vi "Main v00a.vi"() -> ()   [LabVIEW 2017]
uses:
  Controles/Objetos.ctl
  <vilib>/addons/database/Connection.llb/Conn ObjectReference.ctl
  <vilib>/NI/AMC/Update Message Routing Info.vi
  <vilib>/NI/AMC/Create Multiple Messages.vi
  <vilib>/NI/AMC/Read Termination Message.vi
  <vilib>/NI/AMC/Create Single Message.vi
  <vilib>/NI/AMC/Send Message.vi
  <vilib>/NI/AMC/Globals.vi
  <vilib>/Utility/file.llb/Read Delimited Spreadsheet (string).vi
  Globals/Global.vi
  <vilib>/addons/database/Connection.llb/DB Tools Open Connec (Path).vi
  ALT irMonitor/Gobal/Global variables.vi
  <vilib>/addons/database/NI_Database_API.lvlib
  <vilib>/NI/AMC/AMC.lvlib
panel:
  out "BBDD":bool
  in  "Consulta":bool
  in  "Registrado":string
  in  "Cambiar de usuario":bool
  in  "Jiffy csv":path
  in  "Registrar":bool
  out "error out":errorcluster
  in  "Objetos":T1
  out "DataBase":bool
  # "Contabilizador"
  # "powered by"
  # "Contabilizador v00a"
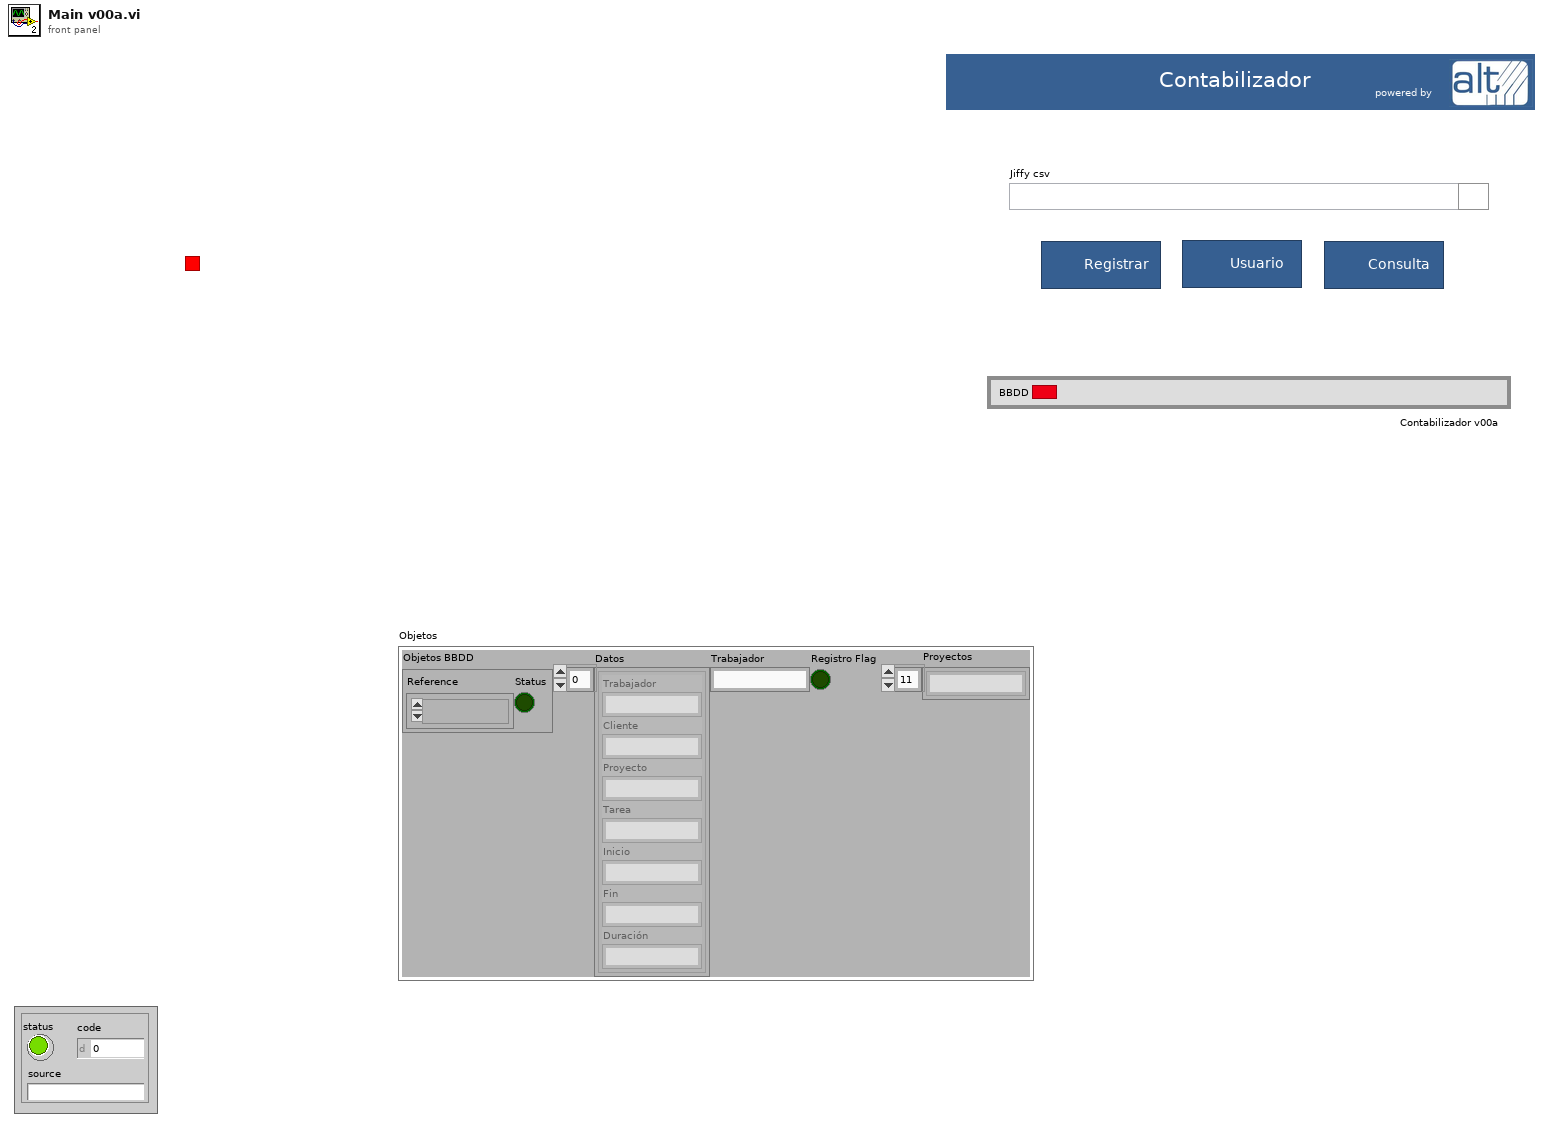
[diagram p1: front panel]
types:
  T1 = typedef "Objetos.ctl" = cluster{"Objetos BBDD":cluster{"Reference":T2, "Status":bool}, "Datos":cluster{"Trabajador":string, "Cliente":string, "Proyecto":string, "Tarea":string, "Inicio":string, "Fin":string, "Duración":string}[], "Trabajador":string, "Registro Flag":bool, "Proyectos":string[]}
  T2 = typedef "NI_Database_API.lvlib/Conn ObjectReference.ctl" = refnum<k1>
  T3 = typedef "AMC.lvlib/Message Queue.ctl" = refnum<queue>
  T4 = cluster{"Trabajador":string, "Cliente":string, "Proyecto":string, "Tarea":string, "Inicio":string, "Fin":string, "Duración":string}
  T5 = cluster{"Nombre de usuario":string, "Contraseña":string, "Trabajador":string}[]
  T6 = cluster{"Trabajador":string, "Cliente":string, "Proyecto":string, "Tarea":string, "Inicio":string, "Fin":string, "Duración":string}[]
  T7 = cluster{"Trabajador":string, "Cliente":string, "Proyecto":string, "Tarea":string, "Inicio":string, "Fin":string, i32}
  T8 = cluster{"Principal":string, "Base de datos":string, "Dialogs":string, "Log":string, "Cam 1":string, "Cam 2":string, "Cam 3":string, "Cam 4":string, "ioLogik":string}
  T9 = cluster{"Nombre":void, "Min":void, "Avg":void, "Max":void, "Condición":void, "Resultado":void, "date/time string":string}
  T10 = cluster{"Database UDL":path, "Settings":path, "Ports":path, "Log Events":path}
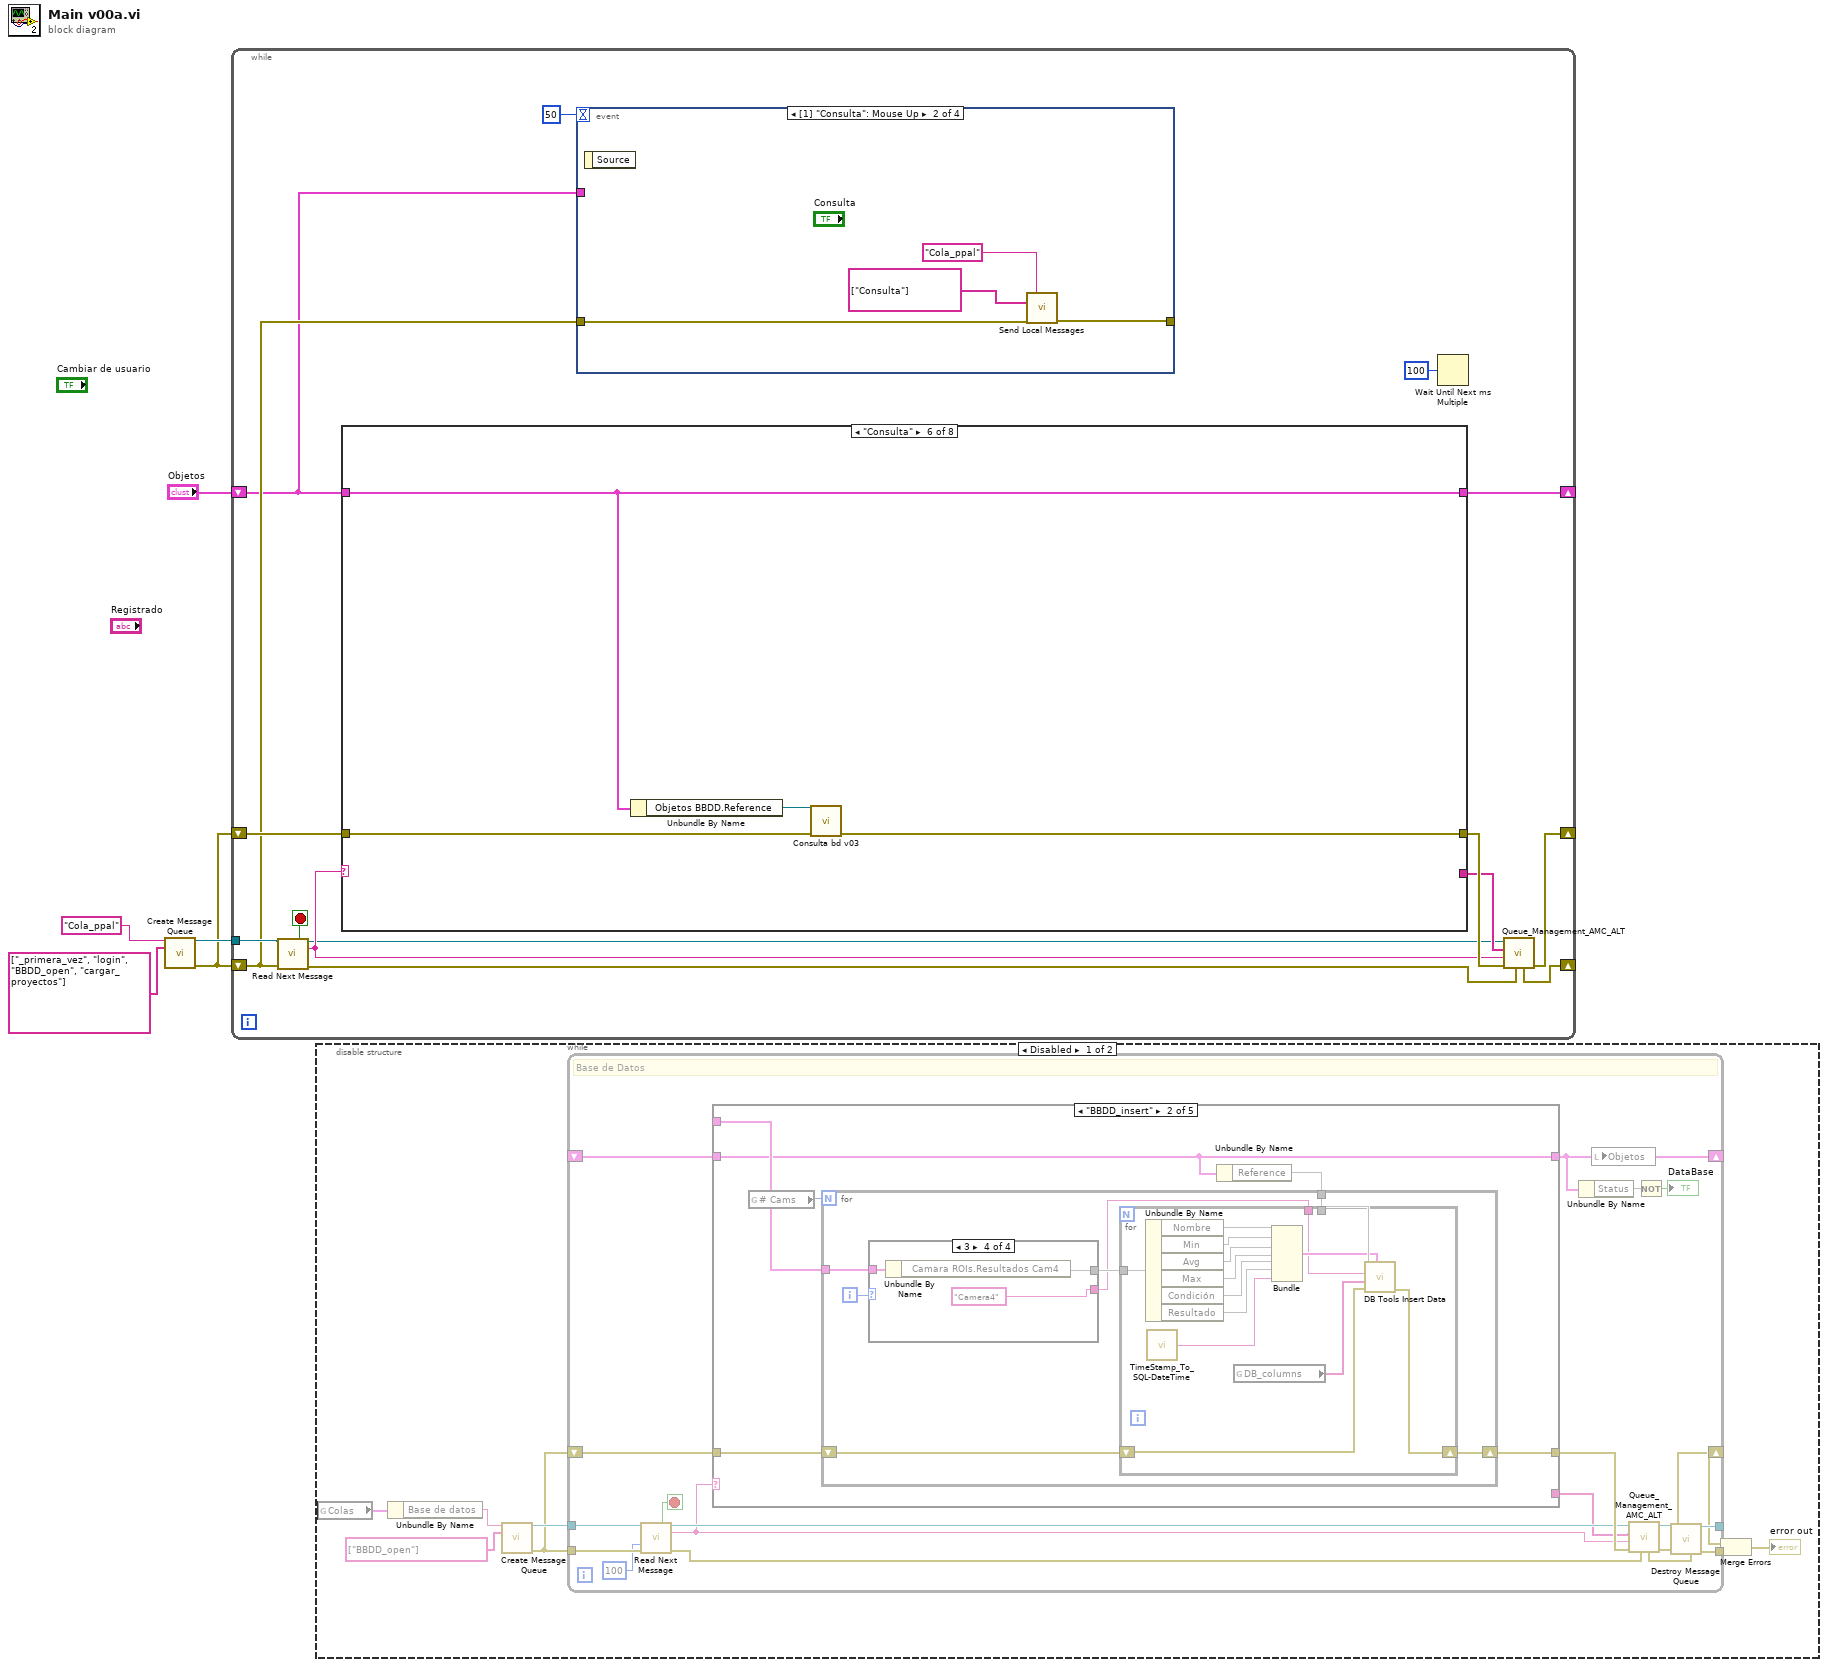
[diagram p0: block diagram]
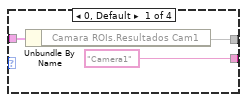
[diagram p3: hidden frame]
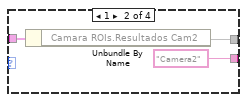
[diagram p4: hidden frame]
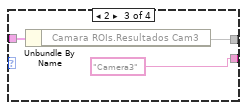
[diagram p5: hidden frame]
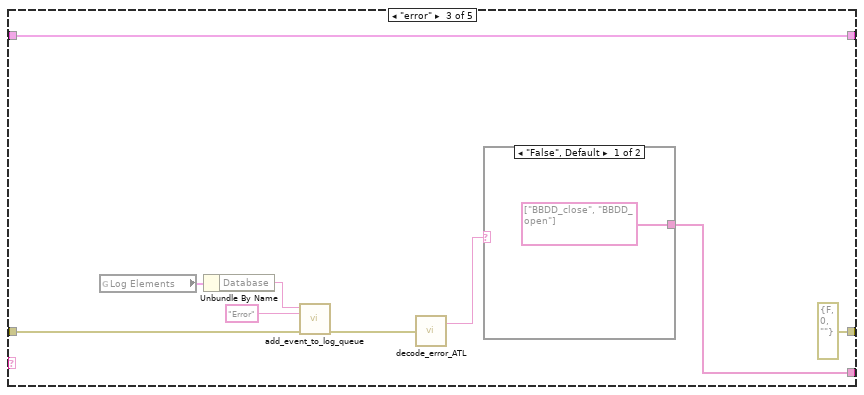
[diagram p6: hidden frame]
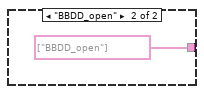
[diagram p7: hidden frame]
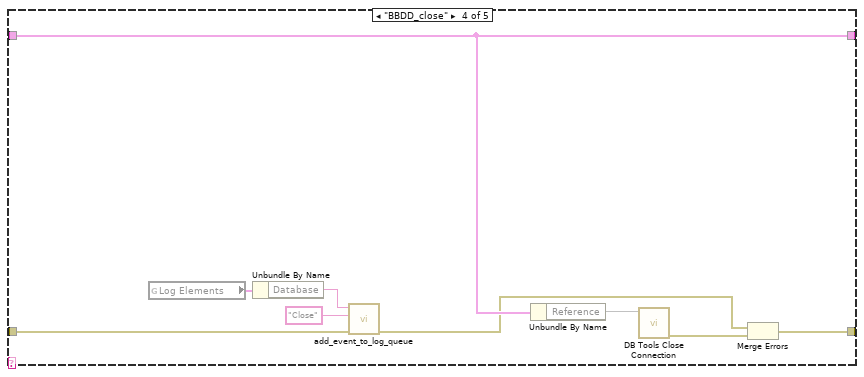
[diagram p8: hidden frame]
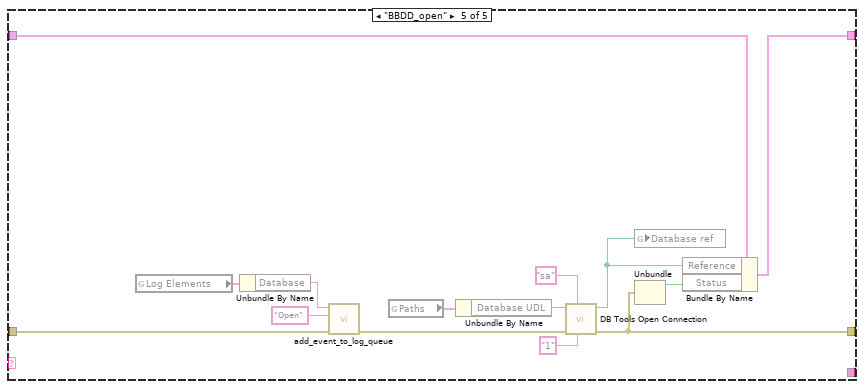
[diagram p9: hidden frame]
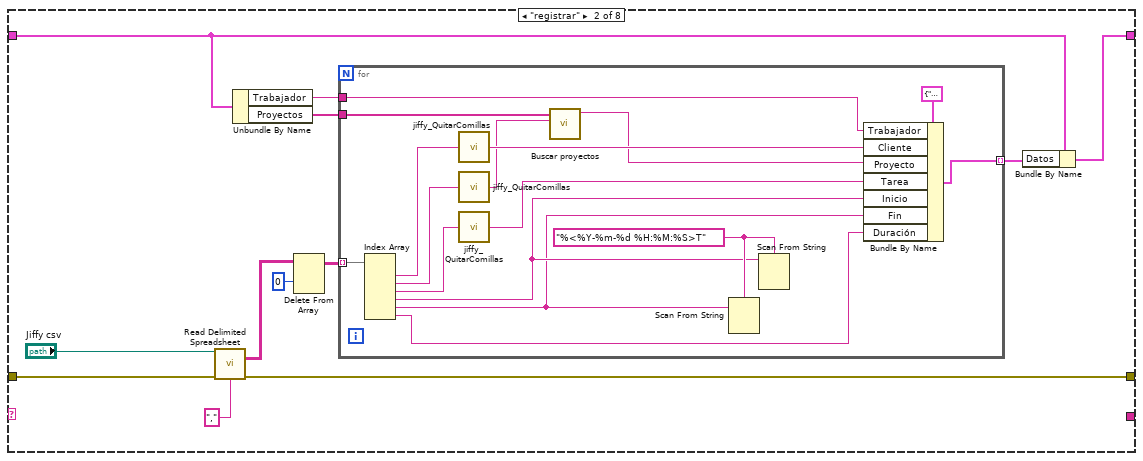
[diagram p12: hidden frame]
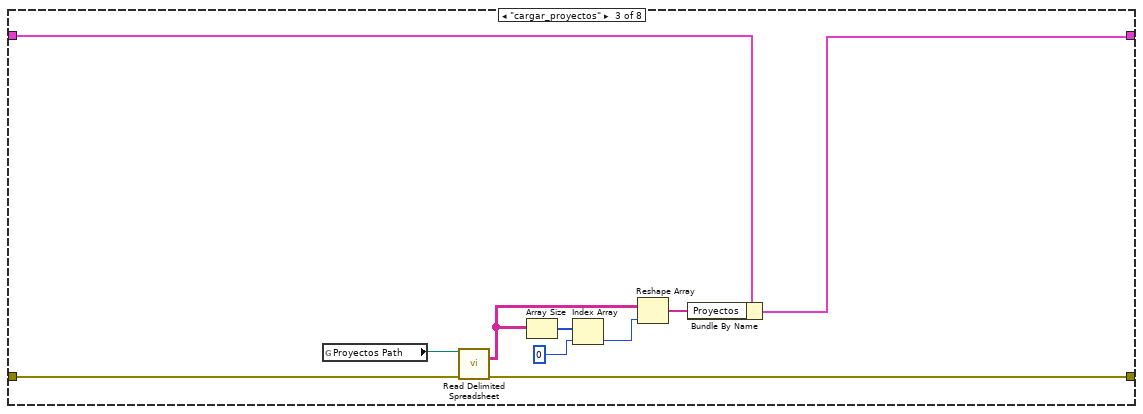
[diagram p13: hidden frame]
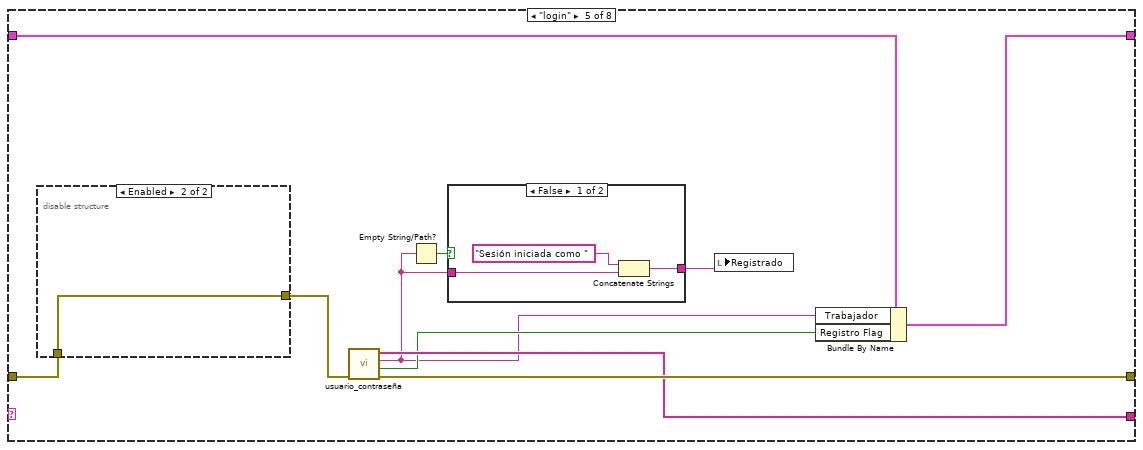
[diagram p15: hidden frame]
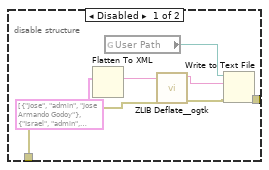
[diagram p16: hidden frame]
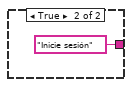
[diagram p17: hidden frame]
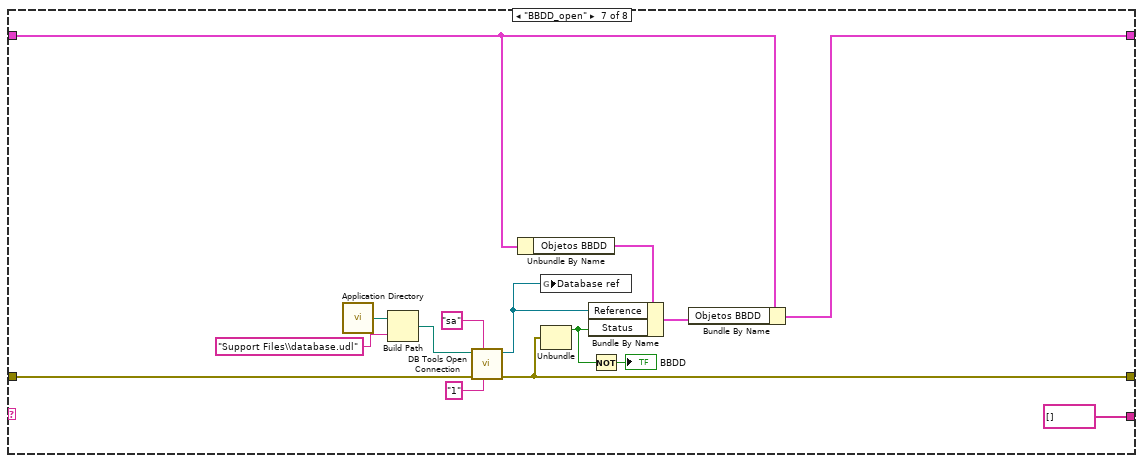
[diagram p18: hidden frame]
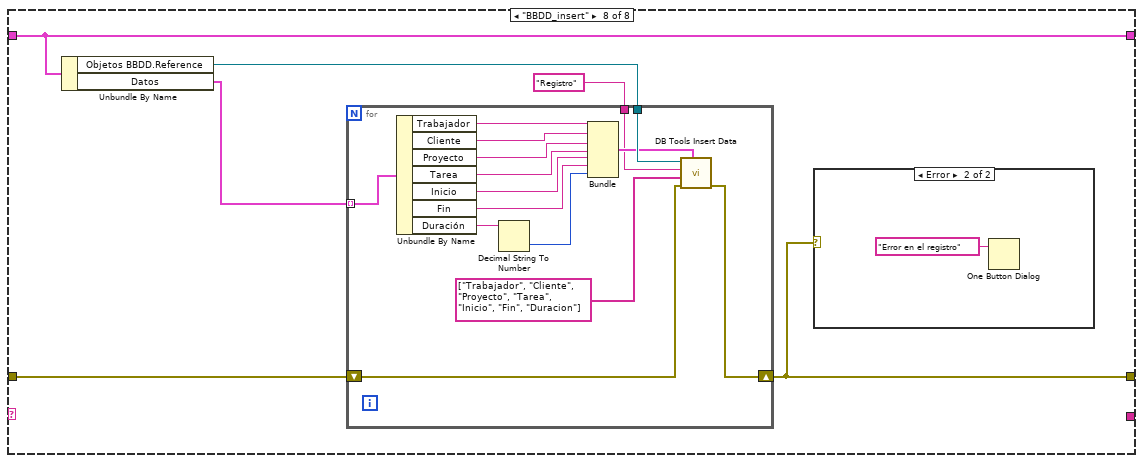
[diagram p19: hidden frame]
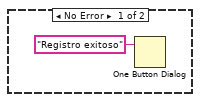
[diagram p20: hidden frame]
diagram:
  n1 = call <vilib>:"Create Message Queue.vi"("message queue name"="Cola_ppal", "initial message names"=string[] ["_primera_vez", "login", "BBDD_open", "cargar_proyectos"]) -> ("message queue out"=w4:T3, "error out"=w1:errorcluster)  [unwired: 12 in]
  n2 = while {
    shift-right: [w17] -> _
    shift-left: w1 -> [w9]
    tunnel: w4 -> [w19]
    shift-right: [w16] -> _
    shift-left: "Objetos" -> [w7]
    shift-right: [w13] -> _
    shift-left: w1 -> [w14]
    stop <- w20 stop-if-true
    n3 = call <vilib>:"Read Next Message.vi"("message queue in"=w19, "error in"=w9) -> ("exit process?"=w20:bool, "message queue out"=w10:T3, "message name"=w11:string, "error out"=w18:errorcluster)  [unwired: 6 in, 4 out]
    n4 = case shown="\"Consulta\"" w11 {
      tunnel: w7 -> [w21 w29 w56 w61 w68 w85 w96 w107]
      tunnel: [w21 w33 w55 w61 w67 w85 w95 w107] -> w16
      tunnel: w14 -> [_ w32 w59 w60 w71 w87 w94 w108]
      tunnel: [_ w31 w58 w60 w70 w86 w93 w103] -> w15
      tunnel: [_ _ _ _ w66 _ string[] [] ("Elementos a cola") _] -> w12
      frame "False", Default {
      }
      frame "registrar" {
        n5 = call-poly <vilib>:"Read Delimited Spreadsheet.vi"("file path (dialog if empty)"="Jiffy csv", "error in (no error)"=w32, "delimiter (\\t)"="," ("delimiter (\\t)")) -> ("all rows"=w27:string[][], "error out"=w31:errorcluster)  [unwired: 7 in, 4 out]
        n6 = Unbundle By Name(w29) -> ("Trabajador"=w23:string, "Proyectos"=w22:string[])
        n7 = Delete From Array(array=w27, index (row)=0) -> (array with subset deleted=w26:string[][])  [unwired: 2 in, 1 out]
        n8 = for {
          tunnel: w26 -> [w49] mode=indexing
          tunnel: [w39] -> w24 mode=indexing
          tunnel: w23 -> [w37]
          tunnel: w22 -> [w35]
          w46 = "%<%Y-%m-%d %H:%M:%S>T" ("format string")
          n9 = Index Array(array=w49) -> (element #1=w45:string, element #2=w48:string, element #3=w47:string, element #4=w41:string, element #5=w40:string, element #6=w38:string)  [unwired: 6 in]
          n10 = call "jiffy_QuitarComillas.vi"("String in"=w45) -> ("String out"=w43:string)
          n11 = call "jiffy_QuitarComillas.vi"("String in"=w48) -> ("String out"=w36:string)
          n12 = call "jiffy_QuitarComillas.vi"("String in"=w47) -> ("String out"=w42:string)
          n13 = call "Buscar proyectos.vi"("String out"=w36, "Proyectos"=w35) -> ("Proyecto"=w34:string)  [unwired: 9 in]
          n14 = Scan From String(format string=w46, input string=w40) -> ()  [unwired: 4 in, 3 out]
          n15 = Scan From String(format string=w46, input string=w41) -> ()  [unwired: 4 in, 3 out]
          n16 = Bundle By Name(cluster=T4 {"Trabajador"="", "Cliente"="", "Proyecto"="", "Tarea"="", "Inicio"="", "Fin"="", "Duración"=""} ("Cluster"), "Trabajador"=w37, "Cliente"=w43, "Proyecto"=w34, "Tarea"=w42, "Inicio"=w41, "Fin"=w40, "Duración"=w38) -> (w39:T4)
        }
        n17 = Bundle By Name(cluster=w29, "Datos"=w24) -> (w33:T1)
      }
      frame "cargar_proyectos" {
        n18 = global read "Global.vi" "Proyectos Path"() -> (w57:path)
        n19 = call-poly <vilib>:"Read Delimited Spreadsheet.vi"("file path (dialog if empty)"=w57, "error in (no error)"=w59) -> ("all rows"=w53:string[][], "error out"=w58:errorcluster)  [unwired: 8 in, 4 out]
        n20 = Array Size(array=w53) -> (size(s)=w52:i32[])
        n21 = Index Array(array=w52, index=0) -> (element=w50:i32)
        n22 = Reshape Array(w53, w50) -> (w54:string[])
        n23 = Bundle By Name(cluster=w56, "Proyectos"=w54) -> (w55:T1)
      }
      frame "_primera_vez" {
      }
      frame "login" {
        n24 = disable-structure shown="Enabled" {
          disable-tunnel: w71 -> [w78 w79]
          disable-tunnel: [w77 w79] -> w69
          frame Disabled {
            n25 = Flatten To XML(anything=T5 [{"Nombre de usuario"="Jose", "Contraseña"="admin", "Trabajador"="Jose Armando Godoy"}, {"Nombre de usuario"="Israel", "Contraseña"="admin", "Trabajador"="Israel Garcia"}, {"Nombre de usuario"="Alejandro", "Contraseña"="admin", "Trabajador"="Alejandro Ortiz"}, {"Nombre de usuario"="Jair", "Contraseña"="admin", "Trabajador"="Jair Paredes"}] ("Array")) -> (xml string=w73:string)
            n26 = global read "Global.vi" "User Path"() -> (w72:path)
            n27 = call <userlib>:"ZLIB Deflate__ogtk.vi"("error in (no error)"=w78, "input"=w73) -> ("error out"=w75:errorcluster, "deflated output"=w76:string)  [unwired: 3 in, 1 out]
            n28 = Write to Text File(file (use dialog)=w72, text=w76, error in=w75) -> (error out=w77:errorcluster)  [unwired: 1 in, 2 out]
          }
          frame Enabled {
          }
        }
        n29 = call "usuario_contraseña.vi"("error in"=w69) -> ("error out"=w70:errorcluster, "Registro Flag"=w65:bool, "Trabajador"=w62:string, "Elemento a cola"=w66:string[])  [unwired: 7 in]
        n30 = Empty String/Path?(string/path=w62) -> (empty?=w64:bool)
        n31 = case shown="False" w64 {
          tunnel: [w81 "Inicie sesión"] -> w63
          tunnel: w62 -> [w80 _]
          frame False {
            n32 = Concatenate Strings("Sesión iniciada como ", w80) -> (w81:string)
          }
          frame True {
          }
        }
        n33 = local write "Registrado"(w63) -> ()
        n34 = Bundle By Name(cluster=w68, "Trabajador"=w62, "Registro Flag"=w65) -> (w67:T1)
      }
      frame "Consulta" {
        n35 = Unbundle By Name(w85) -> ("Objetos BBDD.Reference"=w84:T2)
        n36 = call "Consulta bd v03.vi"("error in (no error)"=w87, "Database"=w84) -> ("error out"=w86:errorcluster)  [unwired: 9 in]
      }
      frame "BBDD_open" {
        n37 = call <vilib>:"Application Directory.vi"() -> ("Application Directory"=w92:path)
        n38 = Build Path(base path=w92, name or relative path="Support Files\\database.udl") -> (appended path=w90:path)
        n39 = call-poly <vilib>:"DB Tools Open Connection.vi"("password"="1", "userID"="sa", "error in (no error)"=w94, "connection information"=w90) -> ("error out"=w93:errorcluster, "connection reference"=w99:T2)  [unwired: 4 in]
        n40 = Unbundle By Name(w96) -> ("Objetos BBDD"=w98:cluster{"Reference":T2, "Status":bool})
        n41 = global write "Global variables.vi" "Database ref"(w99) -> ()
        n42 = Unbundle(w93) -> ("status"=w100:bool)  [unwired: 2 out]
        n43 = Bundle By Name(cluster=w98, "Reference"=w99, "Status"=w100) -> (w97:cluster{"Reference":T2, "Status":bool})
        n44 = Not(x=w100) -> (.not. x?=→"BBDD":bool)
        n45 = Bundle By Name(cluster=w96, "Objetos BBDD"=w97) -> (w95:T1)
      }
      frame "BBDD_insert" {
        n46 = Unbundle By Name(w107) -> ("Objetos BBDD.Reference"=w105:T2, "Datos"=w106:T6)
        n47 = for {
          tunnel: w106 -> [w125] mode=indexing
          tunnel: w105 -> [w123]
          shift-right: [w116] -> w103
          shift-left: w108 -> [w117]
          tunnel: "Registro" ("table") -> [w114]
          n48 = Unbundle By Name(w125) -> ("Trabajador"=w124:string, "Cliente"=w118:string, "Proyecto"=w119:string, "Tarea"=w120:string, "Inicio"=w121:string, "Fin"=w115:string, "Duración"=w113:string)
          n49 = Decimal String To Number(string=w113) -> (number=w112:i32)  [unwired: 2 in, 1 out]
          n50 = Bundle("Trabajador"=w124, "Cliente"=w118, "Proyecto"=w119, "Tarea"=w120, "Inicio"=w121, "Fin"=w115, w112) -> (w122:T7)  [unwired: 1 in]
          n51 = call <vilib>:"DB Tools Insert Data.vi"("data"=w122, "error in (no error)"=w117, "columns"=string[] ["Trabajador", "Cliente", "Proyecto", "Tarea", "Inicio", "Fin", "Duracion"], "table"=w114, "connection reference"=w123) -> ("error out"=w116:errorcluster)  [unwired: 5 in, 1 out]
        }
        n52 = case shown="Error" w103 {
          frame No Error {
            n53 = One Button Dialog(message="Registro exitoso") -> ()  [unwired: 1 in, 1 out]
          }
          frame Error {
            n54 = One Button Dialog(message="Error en el registro") -> ()  [unwired: 1 in, 1 out]
          }
        }
      }
    }
    n55 = event shown="[1] \"Consulta\": Mouse Up" {
      selector: _ -> [_ _ _ _]
      dyn-events: _ -> [_ _ _ _]
      timeout: 50 -> [_ _ _ _]
      tunnel: w9 -> [w126 w127 w132 w138]
      tunnel: [w126 w128 w131 w137] -> _
      tunnel: w7 -> [_ _ _ w136]
      event Timeout {
        n56 = event-data() -> ()  [unwired: 1 in, 3 out]
      }
      event "Consulta": Mouse Up {
        n57 = event-data() -> ()  [unwired: 1 in, 1 out]
        n58 = call <vilib>:"Send Local Messages.vi"("receiver process (\"\" - local)"="Cola_ppal" ("receiver process (\"\" - local)"), "message names"=string[] ["Consulta"] ("message name"), "error in"=w127) -> ("error out"=w128:errorcluster)  [unwired: 10 in, 2 out]
      }
      event "Cambiar de usuario": Mouse Up {
        n59 = event-data() -> ()  [unwired: 1 in, 8 out]
        n60 = call <vilib>:"Send Local Messages.vi"("receiver process (\"\" - local)"="Cola_ppal" ("receiver process (\"\" - local)"), "message names"=string[] ["login"] ("message name"), "error in"=w132) -> ("error out"=w131:errorcluster)  [unwired: 10 in, 2 out]
      }
      event "Registrar": Value Change {
        n61 = event-data() -> ()  [unwired: 1 in, 1 out]
        n62 = Unbundle By Name(w136) -> ("Registro Flag"=w135:bool)
        n63 = case shown="False" w135 {
          tunnel: w138 -> [w140 w143]
          tunnel: [w140 w142] -> w137
          frame False {
            n64 = One Button Dialog(message="Inicie sesión") -> ()  [unwired: 1 in, 1 out]
          }
          frame True {
            n65 = call <vilib>:"Send Local Messages.vi"("receiver process (\"\" - local)"="Cola_ppal" ("receiver process (\"\" - local)"), "message names"=string[] ["registrar", "BBDD_insert"] ("message name"), "error in"=w143) -> ("error out"=w142:errorcluster)  [unwired: 10 in, 2 out]
          }
        }
      }
    }
    n66 = Wait Until Next ms Multiple(millisecond multiple=u32 100) -> ()  [unwired: 1 out]
    n67 = call "Queue_Management_AMC_ALT.vi"("queue error in"=w18, "system error in"=w15, "Case"=w11, "Elementos a cola"=w12, "message queue in"=w10) -> ("system error out"=w13:errorcluster, "queue error out"=w17:errorcluster)  [unwired: 3 in, 2 out]
  }
  n68 = disable-structure shown="Disabled" {
    frame Disabled {
      n69 = global read "Global variables.vi" "Colas"() -> (w146:T8)
      n70 = Unbundle By Name(w146) -> ("Base de datos"=w145:string)
      n71 = call <vilib>:"Create Message Queue.vi"("message queue name"=w145, "initial message names"=string[] ["BBDD_open"]) -> ("message queue out"=w153:T3, "error out"=w152:errorcluster)  [unwired: 12 in]
      n72 = while {
        tunnel: w153 -> [w171]
        tunnel: w152 -> [w170]
        shift-right: [w158] -> _
        shift-left: _ -> [w168]
        shift-right: [w166] -> w148
        shift-left: w152 -> [w169]
        tunnel: [w161] -> w151
        tunnel: [w160] -> w150
        stop <- w155 stop-if-true
        # "Base de Datos"
        n73 = call <vilib>:"Read Next Message.vi"("message queue in"=w171, "timeout (1 ms)"=100, "error in"=w170) -> ("exit process?"=w155:bool, "message queue out"=w164:T3, "message name"=w162:string, "error out"=w163:errorcluster)  [unwired: 5 in, 4 out]
        n74 = case shown="\"BBDD_insert\"" w162 {
          tunnel: w169 -> [w172 w178 w217 w227 w239]
          tunnel: w168 -> [w173 w175 w220 w231 w244]
          tunnel: [w173 w175 w220 w231 w243] -> w158
          tunnel: [w172 w177 errorcluster {"status"=FALSE, "code"=0, "source"=""} ("error out") w229 w240] -> w165
          tunnel: _ -> [_ w176 _ _ _]
          tunnel: [_ _ w218 _ _] -> w159
          frame "Timeout", Default {
          }
          frame "BBDD_insert" {
            n75 = global read "Global variables.vi" "# Cams"() -> (w174:i32)
            n76 = Unbundle By Name(w175) -> ("Reference"=w179)
            n77 = for {
              N: w174 -> [_]
              tunnel: w179 -> [w186]
              shift-right: [w184] -> w177
              shift-left: w178 -> [w185]
              tunnel: w176 -> [w181]
              i -> [w183]
              n78 = case shown="3" w183 {
                tunnel: [w189 w192 w195 w198] -> w182
                tunnel: w181 -> [w188 w191 w194 w197]
                tunnel: ["Camera1" ("table") "Camera2" ("table") "Camera3" ("table") "Camera4" ("table")] -> w180
                frame 0, Default {
                  n79 = Unbundle By Name(w188) -> ("Camara ROIs.Resultados Cam1"=w189)
                }
                frame 1 {
                  n80 = Unbundle By Name(w191) -> ("Camara ROIs.Resultados Cam2"=w192)
                }
                frame 2 {
                  n81 = Unbundle By Name(w194) -> ("Camara ROIs.Resultados Cam3"=w195)
                }
                frame 3 {
                  n82 = Unbundle By Name(w197) -> ("Camara ROIs.Resultados Cam4"=w198)
                }
              }
              n83 = for {
                tunnel: w182 -> [w212]
                tunnel: w186 -> [w210]
                shift-right: [w203] -> w184
                shift-left: w185 -> [w204]
                tunnel: w180 -> [w200]
                n84 = Unbundle By Name(w212) -> ("Nombre"=w211, "Min"=w205, "Avg"=w206, "Max"=w207, "Condición"=w208, "Resultado"=w202)
                n85 = call "TimeStamp_To_SQL-DateTime.vi"() -> ("date/time string"=w201:string)  [unwired: 1 in]
                n86 = global read "Global variables.vi" "DB_columns"() -> (w199:string[])
                n87 = Bundle("Nombre"=w211, "Min"=w205, "Avg"=w206, "Max"=w207, "Condición"=w208, "Resultado"=w202, "date/time string"=w201) -> (w209:T9)  [unwired: 1 in]
                n88 = call <vilib>:"DB Tools Insert Data.vi"("data"=w209, "error in (no error)"=w204, "columns"=w199, "table"=w200, "connection reference"=w210) -> ("error out"=w203:errorcluster)  [unwired: 5 in, 1 out]
              }
            }
          }
          frame "error" {
            n89 = global read "Global variables.vi" "Log Elements"() -> (w215:cluster{"Database":string, "Moxa":string})
            n90 = Unbundle By Name(w215) -> ("Database"=w214:string)
            n91 = call "add_event_to_log_queue.vi"("error in (no error)"=w217, "Evento"="Error", "Elemento"=w214) -> ("error out"=w216:errorcluster)  [unwired: 8 in]
            n92 = call "decode_error_ATL.vi"("error in (no error)"=w216) -> ("case"=w219:string)  [unwired: 1 out]
            n93 = case shown="\"False\", Default" w219 {
              tunnel: [string[] ["BBDD_close", "BBDD_open"] ("message names") string[] ["BBDD_open"] ("message names")] -> w218
              frame "False", Default {
              }
              frame "BBDD_open" {
              }
            }
          }
          frame "BBDD_close" {
            n94 = global read "Global variables.vi" "Log Elements"() -> (w228:cluster{"Database":string, "Moxa":string})
            n95 = Unbundle By Name(w228) -> ("Database"=w225:string)
            n96 = call "add_event_to_log_queue.vi"("error in (no error)"=w227, "Evento"="Close", "Elemento"=w225) -> ("error out"=w226:errorcluster)  [unwired: 8 in]
            n97 = Unbundle By Name(w231) -> ("Reference"=w232)
            n98 = call <vilib>:"DB Tools Close Connection.vi"("connection reference"=w232) -> ("error out"=w230:errorcluster)  [unwired: 6 in]
            n99 = Merge Errors(w226, w230) -> (w229:errorcluster)
          }
          frame "BBDD_open" {
            n100 = global read "Global variables.vi" "Log Elements"() -> (w237:cluster{"Database":string, "Moxa":string})
            n101 = Unbundle By Name(w237) -> ("Database"=w234:string)
            n102 = call "add_event_to_log_queue.vi"("error in (no error)"=w239, "Evento"="Open", "Elemento"=w234) -> ("error out"=w238:errorcluster)  [unwired: 8 in]
            n103 = global read "Global variables.vi" "Paths"() -> (w236:T10)
            n104 = Unbundle By Name(w236) -> ("Database UDL"=w235:path)
            n105 = call-poly <vilib>:"DB Tools Open Connection.vi"("password"="1", "userID"="sa", "error in (no error)"=w238, "connection information"=w235) -> ("error out"=w240:errorcluster, "connection reference"=w241:T2)  [unwired: 4 in]
            n106 = global write "Global variables.vi" "Database ref"(w241) -> ()
            n107 = Unbundle(w240) -> ("status"=w242:bool)  [unwired: 2 out]
            n108 = Bundle By Name(cluster=w244, "Reference"=w241, "Status"=w242) -> (w243:cluster{})
          }
        }
        n109 = Unbundle By Name(w158) -> ("Status"=w157)
        n110 = local write "Objetos"(w158) -> ()
        n111 = call "Queue_Management_AMC_ALT.vi"("queue error in"=w163, "system error in"=w165, "Case"=w162, "Elementos a cola"=w159, "message queue in"=w164) -> ("system error out"=w166:errorcluster, "message queue out"=w161:T3, "queue error out"=w160:errorcluster)  [unwired: 3 in, 1 out]
        n112 = Not(x=w157) -> (.not. x?=→"DataBase":bool)
      }
      n113 = call <vilib>:"Destroy Message Queue.vi"("message queue in"=w151, "error in"=w150) -> ("error out"=w149:errorcluster)  [unwired: 11 in, 2 out]
      n114 = Merge Errors(w148, w149) -> (→"error out":errorcluster)
    }
    frame Enabled {
    }
  }
